vi "Launcher - TopUI.vi"(6 "Worker Alias":string="TopUI", 8 "error in":errorcluster, 9 "Initialization Data":T1, 11 "TopUI in":refnum<class "TopUI.lvclass">) -> (0 "error out":errorcluster)   [LabVIEW 2025]
doc: "This VI launches the Head Worker of a Workers application."
uses:
  Workers/TopUI/Initialization Data.ctl
  Workers/TopUI/Response Cases.ctl
  Workers/TopUI/TopUI.lvclass
  ScopeAA/ScopeAA.lvclass
  ScopeBB/ScopeBB.lvclass
  Workers/TopUI/TopUI.lvclass/TopUI.ctl
  Workers/TopUI/Write Oscilloscope.vi
  <vilib>/addons/_Workers/Debugger/Debug Client/Debug Client.lvlib
panel:
  in  "ClassSelect":enum16{"ScopeAA", "ScopeBB"}(ring)
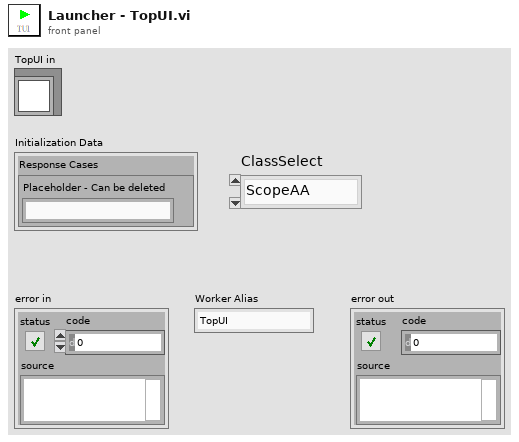
[diagram p1: front panel]
types:
  T1 = typedef "TopUI.lvclass/Initialization Data.ctl" = cluster{"Response Cases":T2}
  T2 = typedef "TopUI.lvclass/Response Cases.ctl" = cluster{"Placeholder - Can be deleted":string}
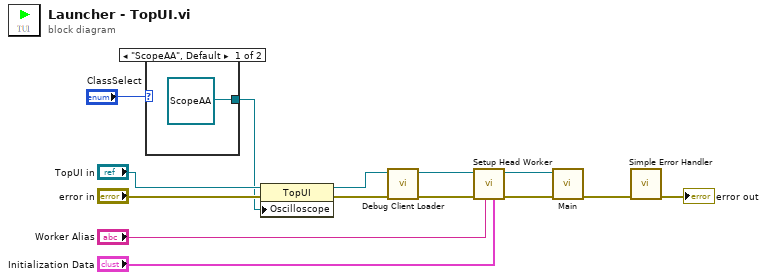
[diagram p0: block diagram]
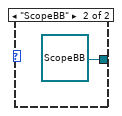
[diagram p2: hidden frame]
diagram:
  n1 = case shown="\"ScopeAA\", Default" "ClassSelect" {
    tunnel: [refnum<class "ScopeAA.lvclass"> refnum ("ScopeAA.lvclass") refnum<class "ScopeBB.lvclass"> refnum ("ScopeBB.lvclass")] -> w1
    frame "ScopeAA", Default {
    }
    frame "ScopeBB" {
    }
  }
  n2 = property class="TopUI"(reference="TopUI in", error in="error in", "Oscilloscope"=w1) -> (reference out=w3:refnum<class "TopUI.lvclass">, error out=w5:errorcluster)
  n3 = call <vilib>:"Debug Client Loader.vi"("error in (no error)"=w5, "Worker_"=w3) -> ("error out"=w7:errorcluster, "Worker_out"=w6:refnum<class "TopUI.lvclass">)  [unwired: 8 in]
  n4 = call-dynamic "Setup Head Worker.vi"("Initalization Data"="Initialization Data", "Worker Alias"="Worker Alias", "error in"=w7, "Worker_"=w6) -> ("error out"=w14:errorcluster, "Worker_out"=w11:refnum<class "TopUI.lvclass">)  [unwired: 6 in]
  n5 = call-dynamic "Main.vi"("error in"=w14, "TopUI in"=w11) -> ("error out"=w12:errorcluster)  [unwired: 8 in, 1 out]
  n6 = call <vilib>:"Simple Error Handler.vi"("error in (no error)"=w12) -> ("error out"=→"error out":errorcluster)  [unwired: 4 in, 4 out]
